vi "SetZeroFCG.vi"(8 "error in (no error)":errorcluster) -> (0 "error out":errorcluster)   [LabVIEW 2011]
uses:
  Variables/GlobalSetGetConfigureCamera.vi
  Variables/ccdChipPixels.vi
  Variables/GlobalSetGetHeidenhainParameters.vi
  Variables/GlobalSetNumberOfDigits_PhysikalInstruments.vi
  Variables/405Pico.vi
  Variables/625CubeLaser.vi
  Variables/GlobalGetMesaurementStatus.vi
  Variables/GlobalExitVar.vi
  Variables/GrapRoi.vi
  Variables/GlobalGetPhysikalInstrumentsOnOff.vi
  Variables/StartStopMesaurement.vi
  Variables/GlobalLaserEmissionOnOffInterlook.vi
  Variables/GlobalGetHeidenhainDriftOnOff.vi
  Variables/GlobalGetConfigurationStatus.vi
  Variables/GlobalGetInitialisationStatus.vi
  Variables/GlobalGetKoherasLaserOnOff.vi
  Variables/GlobalGetAOTFOnOff.vi
  Variables/GlobalGetAvantesSpectrometerOnOff.vi
  Variables/GlobalGetCamerasOnOff.vi
  Variables/SetRoi.vi
  Variables/GetPicture.vi
  Variables/StopGetPic.vi
  Variables/GlobalSetGetParametersAvantes.vi
  Variables/GlobalSetGetPositionParameters.vi
  Variables/GlobalSetGetTriggerForPointMeasurement.vi
  Variables/GlobalSetGetPixelOfRoi.vi
  Variables/GetSetGlobalPath2StoreStackData.vi
  Variables/cameraHandler.vi
  Variables/GlobalCameraDebugTemperature.vi
  Variables/ScannerMirrorStatus.vi
  Variables/GlobalGetSetMeasurementType.vi
  Variables/GlobalSetNumberOfDigits_Scanners.vi
  Variables/AOTF_NonLinearLinesOnOff.vi
  Variables/ModulationNiveaus.vi
  Variables/IlluminationPatterns.vi
  Variables/GlobalImage.vi
  Variables/GlobalGetBeamDiagnostics.vi
  Variables/GlobalStopGetBeamDiagnostics.vi
panel:
  in  "out":T1
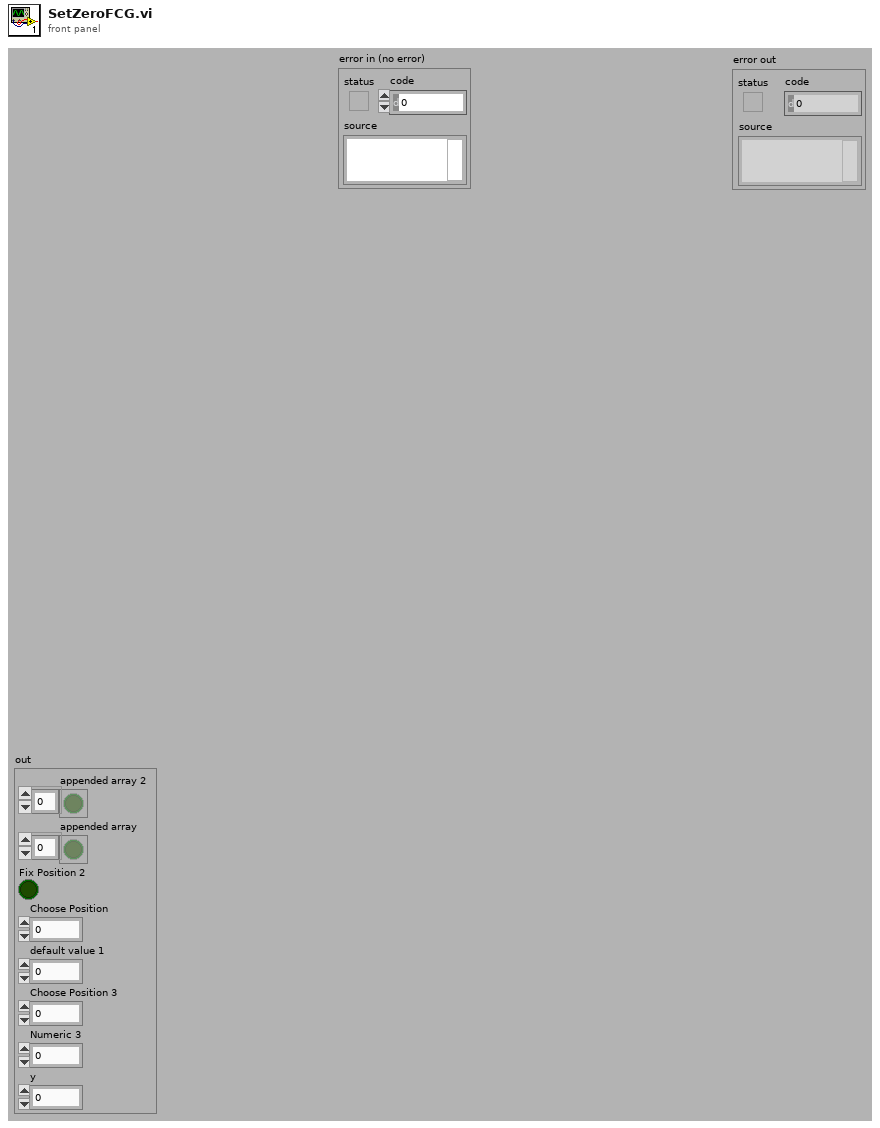
[diagram p1: front panel]
types:
  T1 = cluster{"appended array 2":bool[], "appended array":bool[], "Fix Position 2":bool, "Choose Position":dbl, "default value 1":dbl, "Choose Position 3":dbl, "Numeric 3":i32, "y":i32}
  T2 = enum32{"Non Linear Illumniation", "Constant Illumination"}
  T3 = cluster{"numbers of \nmeasurements":i16, "startPixel":u16, "stopPixel":u16, "intTime / [ms]":sgl, "backgroundSubtract":bool, "numAvg":u32}
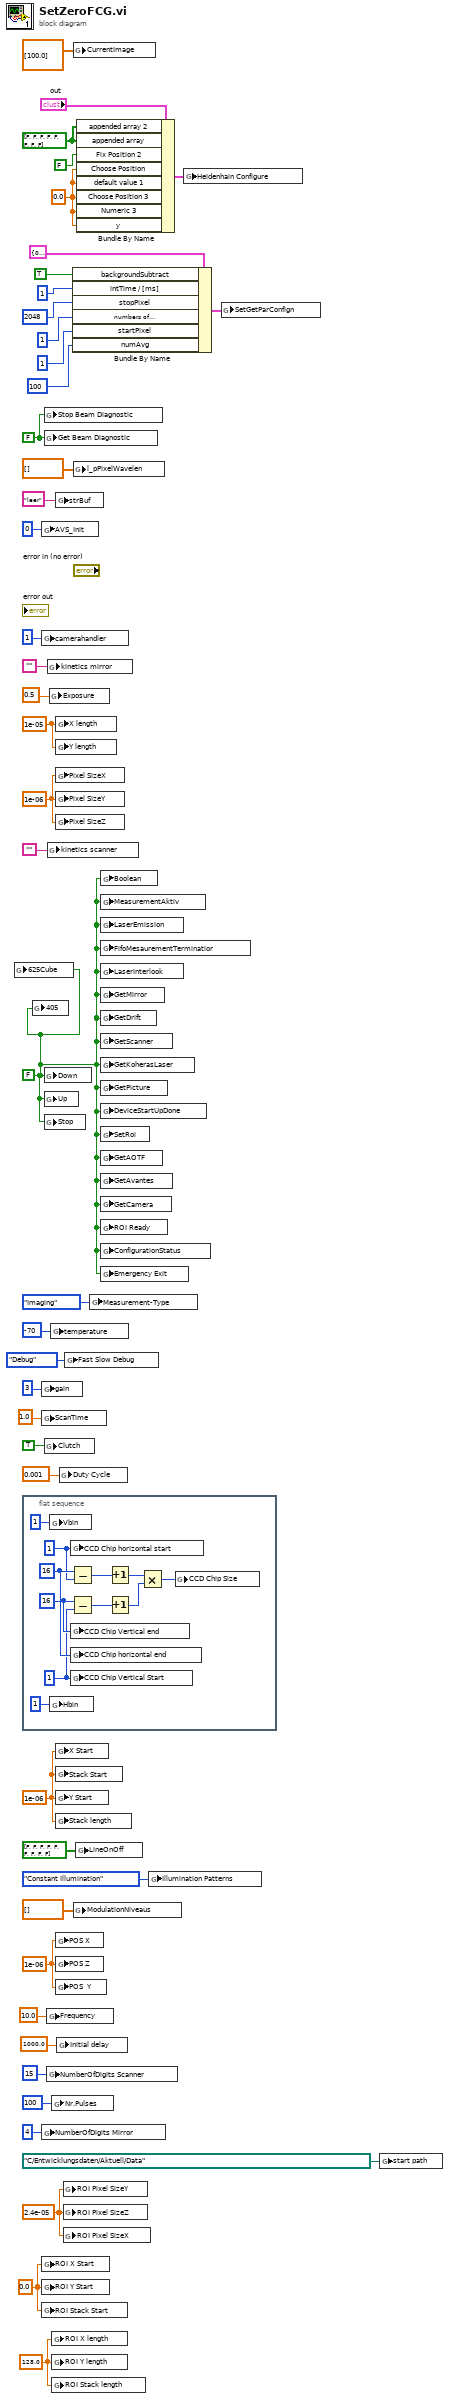
[diagram p0: block diagram]
diagram:
  w3 = FALSE ("Stop Beam Diagnostic")
  w20 = 128.0 ("ROI Stack length")
  w21 = 0.0 ("ROI Stack Start")
  w22 = 2.4e-05 ("ROI Pixel SizeX")
  w16 = 1e-05 ("X length")
  w19 = 1e-06 ("X Start")
  w17 = 1e-06 ("Pixel SizeX")
  w31 = 1e-06 ("Duty Cycle")
  w1 = FALSE ("andor 2")
  w44 = 0.0 ("Choose Position")
  w45 = bool[] [FALSE, FALSE, FALSE, FALSE, FALSE, FALSE, FALSE, FALSE] ("appended array")
  n1 = global write "625CubeLaser.vi" "625Cube"(w1) -> ()
  n2 = flat-sequence {
    frame #0 {
      w50 = 16 ("CCD Chip Vertical end")
      w47 = 1 ("CCD Chip Vertical Start")
      w49 = 16 ("CCD Chip horizontal end")
      w48 = 1
      n3 = global write "GlobalSetGetConfigureCamera.vi" "Vbin"(1 ("Vbin")) -> ()
      n4 = global write "GlobalSetGetConfigureCamera.vi" "Hbin"(1 ("Hbin")) -> ()
      n5 = Subtract(x=w50, y=w48) -> (x-y=w52:i32)
      n6 = Subtract(x=w49, y=w47) -> (x-y=w51:i32)
      n7 = global write "ccdChipPixels.vi" "CCD Chip horizontal start"(w48) -> ()
      n8 = global write "ccdChipPixels.vi" "CCD Chip Vertical end"(w49) -> ()
      n9 = global write "ccdChipPixels.vi" "CCD Chip horizontal end"(w50) -> ()
      n10 = global write "ccdChipPixels.vi" "CCD Chip Vertical Start"(w47) -> ()
      n11 = Increment(x=w52) -> (x+1=w54:i32)
      n12 = Increment(x=w51) -> (x+1=w53:i32)
      n13 = Multiply(x=w54, y=w53) -> (x*y=w57:i32)
      n14 = global write "ccdChipPixels.vi" "CCD Chip Size"(w57) -> ()
    }
  }
  n15 = global write "405Pico.vi" "405"(w1) -> ()
  n16 = global write "GlobalSetGetParametersAvantes.vi" "AVS_Init"(0 ("AVS_Init")) -> ()
  n17 = global write "cameraHandler.vi" "camerahandler"(1 ("camerahandler")) -> ()
  n18 = global write "GlobalSetGetConfigureCamera.vi" "gain"(3 ("gain")) -> ()
  n19 = global write "GlobalSetGetPositionParameters.vi" "ScanTime"(1.0 ("Duty Cycle")) -> ()
  n20 = global write "GlobalSetNumberOfDigits_PhysikalInstruments.vi" "NumberOfDigits Mirror"(4 ("NumberOfDigits")) -> ()
  n21 = global write "GlobalSetGetPixelOfRoi.vi" "ROI X Start"(w21) -> ()
  n22 = global write "GlobalSetGetPixelOfRoi.vi" "ROI Y Start"(w21) -> ()
  n23 = global write "GlobalSetGetPixelOfRoi.vi" "ROI Stack Start"(w21) -> ()
  n24 = global write "GlobalStopGetBeamDiagnostics.vi" "Stop Beam Diagnostic"(w3) -> ()
  n25 = global write "GlobalGetBeamDiagnostics.vi" "Get Beam Diagnostic"(w3) -> ()
  n26 = global write "GlobalSetGetHeidenhainParameters.vi" "Down"(w1) -> ()
  n27 = global write "GlobalSetGetHeidenhainParameters.vi" "Up"(w1) -> ()
  n28 = global write "StopGetPic.vi" "Stop"(w1) -> ()
  n29 = global write "GlobalSetGetHeidenhainParameters.vi" "Clutch"(TRUE ("Clutch")) -> ()
  n30 = global write "GlobalSetGetTriggerForPointMeasurement.vi" "Frequency"(10.0 ("Frequency")) -> ()
  n31 = global write "GlobalSetNumberOfDigits_Scanners.vi" "NumberOfDigits Scanner"(15 ("NumberOfDigits Scanner")) -> ()
  n32 = global write "ScannerMirrorStatus.vi" "kinetics mirror"("") -> ()
  n33 = global write "ScannerMirrorStatus.vi" "kinetics scanner"("") -> ()
  n34 = global write "GlobalSetGetConfigureCamera.vi" "Exposure"(sgl 0.5 ("ExpTime")) -> ()
  n35 = global write "GlobalCameraDebugTemperature.vi" "temperature"(-70 ("temperature")) -> ()
  n36 = global write "GlobalSetGetTriggerForPointMeasurement.vi" "Nr.Pulses"(100 ("Nr.Pulses")) -> ()
  n37 = global write "GlobalSetGetPixelOfRoi.vi" "ROI X length"(w20) -> ()
  n38 = global write "GlobalSetGetPixelOfRoi.vi" "ROI Y length"(w20) -> ()
  n39 = global write "GlobalSetGetPixelOfRoi.vi" "ROI Stack length"(w20) -> ()
  n40 = global write "GlobalSetGetParametersAvantes.vi" "strBuf"("leer" ("strBuf")) -> ()
  n41 = global write "GlobalSetGetPixelOfRoi.vi" "X length"(w16) -> ()
  n42 = global write "GlobalSetGetPixelOfRoi.vi" "Y length"(w16) -> ()
  n43 = global write "GlobalSetGetPixelOfRoi.vi" "Pixel SizeX"(w17) -> ()
  n44 = global write "GlobalSetGetPixelOfRoi.vi" "Pixel SizeY"(w17) -> ()
  n45 = global write "GlobalSetGetPixelOfRoi.vi" "Pixel SizeZ"(w17) -> ()
  n46 = global write "GlobalSetGetPixelOfRoi.vi" "X Start"(w19) -> ()
  n47 = global write "GlobalSetGetPixelOfRoi.vi" "Stack Start"(w19) -> ()
  n48 = global write "GlobalSetGetPixelOfRoi.vi" "Y Start"(w19) -> ()
  n49 = global write "GlobalSetGetPixelOfRoi.vi" "Stack length"(w19) -> ()
  n50 = global write "GlobalSetGetPositionParameters.vi" "POS X"(w31) -> ()
  n51 = global write "GlobalSetGetPositionParameters.vi" "POS Z"(w31) -> ()
  n52 = global write "GlobalSetGetPositionParameters.vi" "POS  Y"(w31) -> ()
  n53 = global write "GlobalSetGetTriggerForPointMeasurement.vi" "Initial delay"(1000.0 ("Initial delay")) -> ()
  n54 = global write "GlobalSetGetTriggerForPointMeasurement.vi" "Duty Cycle"(0.001 ("Duty Cycle")) -> ()
  n55 = global write "GlobalSetGetPixelOfRoi.vi" "ROI Pixel SizeY"(w22) -> ()
  n56 = global write "GlobalSetGetPixelOfRoi.vi" "ROI Pixel SizeZ"(w22) -> ()
  n57 = global write "GlobalSetGetPixelOfRoi.vi" "ROI Pixel SizeX"(w22) -> ()
  n58 = global write "GlobalCameraDebugTemperature.vi" "Fast Slow Debug"(enum32{"Normal", "Debug"}."Debug" ("Fast Slow Debug")) -> ()
  n59 = Bundle By Name(cluster=T3 {"numbers of \nmeasurements"=0, "startPixel"=0, "stopPixel"=0, "intTime / [ms]"=0.0, "backgroundSubtract"=FALSE, "numAvg"=0} ("out"), "backgroundSubtract"=TRUE, "intTime / [ms]"=u16 1 ("startPixel"), "stopPixel"=u16 2048, "numbers of \nmeasurements"=i16 1 ("numbers of \nmeasurements"), "startPixel"=u16 1, "numAvg"=u32 100) -> (w28:T3)
  n60 = global write "GlobalImage.vi" "CurrentImage"(dbl[][] [[100.0]] ("CurrentImage")) -> ()
  n61 = global write "GlobalSetGetParametersAvantes.vi" "l_pPixelWavelen"(dbl[] [] ("l_pPixelWavelen")) -> ()
  n62 = global write "ModulationNiveaus.vi" "ModulationNiveaus"(dbl[] [] ("ModulationNiveaus")) -> ()
  n63 = global write "AOTF_NonLinearLinesOnOff.vi" "LineOnOff"(bool[] [FALSE, FALSE, FALSE, FALSE, FALSE, FALSE, FALSE, FALSE, FALSE] ("LineOnOff")) -> ()
  n64 = Bundle By Name(cluster="out", "appended array 2"=w45, "appended array"=w45, "Fix Position 2"=FALSE, "Choose Position"=w44, "default value 1"=w44, "Choose Position 3"=w44, "Numeric 3"=w44, "y"=w44) -> (w29:T1)
  n65 = global write "GlobalGetSetMeasurementType.vi" "Measurement-Type"(enum32{"Diffusion", "Imaging"}."Imaging" ("Measurement-Type")) -> ()
  n66 = global write "StartStopMesaurement.vi" "Boolean"(w1) -> ()
  n67 = global write "GlobalGetMesaurementStatus.vi" "MeasurementAktiv"(w1) -> ()
  n68 = global write "GlobalLaserEmissionOnOffInterlook.vi" "LaserEmission"(w1) -> ()
  n69 = global write "GlobalGetMesaurementStatus.vi" "FifoMesaurementTerminatior"(w1) -> ()
  n70 = global write "GlobalLaserEmissionOnOffInterlook.vi" "LaserInterlook"(w1) -> ()
  n71 = global write "GlobalGetPhysikalInstrumentsOnOff.vi" "GetMirror"(w1) -> ()
  n72 = global write "GlobalGetHeidenhainDriftOnOff.vi" "GetDrift"(w1) -> ()
  n73 = global write "GlobalGetPhysikalInstrumentsOnOff.vi" "GetScanner"(w1) -> ()
  n74 = global write "GlobalGetKoherasLaserOnOff.vi" "GetKoherasLaser"(w1) -> ()
  n75 = global write "GetPicture.vi" "GetPicture"(w1) -> ()
  n76 = global write "GlobalGetInitialisationStatus.vi" "DeviceStartUpDone"(w1) -> ()
  n77 = global write "SetRoi.vi" "SetRoi"(w1) -> ()
  n78 = global write "GlobalGetAOTFOnOff.vi" "GetAOTF"(w1) -> ()
  n79 = global write "GlobalGetAvantesSpectrometerOnOff.vi" "GetAvantes"(w1) -> ()
  n80 = global write "GlobalGetCamerasOnOff.vi" "GetCamera"(w1) -> ()
  n81 = global write "GrapRoi.vi" "ROI Ready"(w1) -> ()
  n82 = global write "GlobalGetConfigurationStatus.vi" "ConfigurationStatus"(w1) -> ()
  n83 = global write "GlobalExitVar.vi" "Emergency Exit"(w1) -> ()
  n84 = global write "IlluminationPatterns.vi" "Illumination Patterns"(T2."Constant Illumination" ("Illumination Patterns")) -> ()
  n85 = global write "GlobalSetGetHeidenhainParameters.vi" "Heidenhain Configure"(w29) -> ()
  n86 = global write "GlobalSetGetParametersAvantes.vi" "SetGetParConfign"(w28) -> ()
  n87 = global write "GetSetGlobalPath2StoreStackData.vi" "start path"(path "C:/Entwicklungsdaten/Aktuell/Data" ("start path")) -> ()
